vi "Create from Ref.vi"(6 "TSnax:Engine":refnum<class "Engine.lvclass">, 8 "error in (no error)":errorcluster, 10 "Event Common Data":T1, 11 "msg":refnum<k7>) -> (0 "error out":errorcluster, 2 "Code":T2, 3 "UIMessage out":refnum<class "UIMessage.lvclass">)   [LabVIEW 2020, in "TSnax.lvlib" / "UIMessage.lvclass"]
uses:
  UIMessage.lvclass
  UIMsg.ctl
  Engine/Engine.lvclass
  UIMessage.lvclass/UIMessage.ctl
  TSnax.lvlib
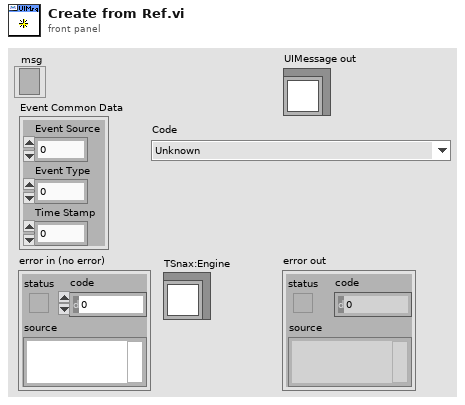
[diagram p1: front panel]
types:
  T1 = cluster{"Event Source":i32, "Event Type":u32, "Time Stamp":u32}
  T2 = typedef "TSnax.lvlib/UIMsg.ctl" = enum16{"Unknown", "BreakOnUserRequest", "BreakOnBreakpoint", "BreakOnRunTimeError", "Trace", "TerminatingExecution", "AbortingExecution", "KillingExecutionThreads", "EndExecution", "ShutDownComplete", "StartExecution", "ProgressPercent", "ProgressText", "StartInteractiveExecution", "EndInteractiveExecution", "TerminatingInteractiveExecution", "TerminationCancelled", "ResumeFromBreak", "StartFileExecution", "EndFileExecution", "ShutDownCancelled", "LocalizationSettingChanged", "OpenWindows", "TileWindows", "CascadeWindows", "ReportChanged", "CloseWindows", "RefreshWindows", "ClientFileChanged", "DisplayReport", "ModelState_Initializing", "ModelState_Waiting", "ModelState_Identified", "ModelState_BeginTesting", "ModelState_TestingComplete", "ModelState_PostProcessingComplete", "ModelState_EnabledStateSet", "ReportLocationChanged", "GotoLocation", "PushUndoItem", "OutputMessages", "TypePaletteFileListChanged", "NonTerminatingThreadsArePreventingTermination", "ModelState_PostProcessing", "ReportCollectionChanged", "RuntimeError"}
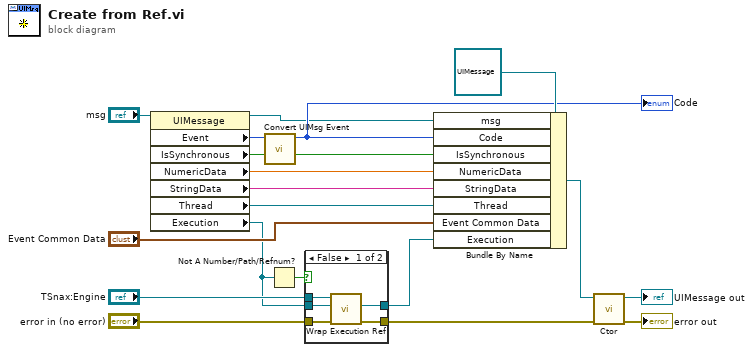
[diagram p0: block diagram]
diagram:
  n1 = property class="UIMessage"(reference="msg") -> (reference out=w11:refnum<k7>, "Event"=w17:i32, "IsSynchronous"=w13:bool, "NumericData"=w14:dbl, "StringData"=w15:string, "Thread"=w16:refnum<k7>, "Execution"=w2:refnum<k7>)  [unwired: 1 in, 1 out]
  n2 = call "Convert UIMsg Event.vi"("UIMsg Event"=w17) -> ("UIMsg"=w12:T2)  [unwired: 9 in, 1 out]
  "Code" <- w12
  n3 = Not A Number/Path/Refnum?(number/path/refnum=w2) -> (NaN/Path/Refnum?=w1:bool)
  n4 = case shown="False" w1 {
    tunnel: "TSnax:Engine" -> [w24 _]
    tunnel: [w23 _] -> w5
    tunnel: "error in (no error)" -> [w22 w25]
    tunnel: [w21 w25] -> w3
    tunnel: w2 -> [w20 _]
    frame False {
      n5 = call "Wrap Execution Ref.vi"("error in (no error)"=w22, "Execution Ref"=w20, "Engine in"=w24) -> ("error out"=w21:errorcluster, "Execution"=w23:refnum<class "Execution.lvclass">)  [unwired: 6 in, 1 out]
    }
    frame True {
    }
  }
  n6 = Bundle By Name(cluster=refnum<class "UIMessage.lvclass"> refnum ("UIMessage in"), "msg"=w11, "Code"=w12, "IsSynchronous"=w13, "NumericData"=w14, "StringData"=w15, "Thread"=w16, "Event Common Data"="Event Common Data", "Execution"=w5) -> (w8:refnum<class "UIMessage.lvclass">)
  n7 = call-dynamic "Ctor.vi"("error in (no error)"=w3, "PropertyObject in"=w8) -> ("error out"=→"error out":errorcluster, "PropertyObject out"=→"UIMessage out":refnum<class "UIMessage.lvclass">)  [unwired: 8 in]
